vi "Image with metadata to Tiff file string.vi"(4 "error in":errorcluster, 5 "Compression Type (None)":i32(ring) items=["None", "JPEG", "Run Length Encoded", "Zip"], 6 "ImageDescription string\n(must be at least 5 char long)":string=" Four score and seven years ago our fathers brought forth on this continent, a new nation, conceived in Liberty, and dedicated to the proposition that all men are created equal.\n\nNow we are engaged in a great civil war, testing whether that nation, or any nation so conceived and so dedicated, can long endure. We are met on a great battle-field of that war. We have come to dedicate a portion of that field, as a final resting place for those who here gave their lives that that nation might live. It is altogether fitting and proper that we should do this.\n\nBut, in a larger sense, we can not dedicate -- we can not consecrate -- we can not hallow -- this ground. The brave men, living and dead, who struggled here, have consecrated it, far above our poor power to add or detract. The world will little note, nor long remember what we say here, but it can never forget what they did here. It is for us the living, rather, to be dedicated here to the unfinished work which they who fought here have thus far so nobly advanced. It is rather for us to be here dedicated to the great task remaining before us -- that from these honored dead we take increased devotion to that cause for which they gave the last full measure of devotion -- that we here highly resolve that these dead shall not have died in vain -- that this nation, under God, shall have a new birth of freedom -- and that government of the people, by the people, for the people, shall not perish from the earth. ", 7 "img":T1) -> (0 "error out":errorcluster, 1 "Time elapsed (ms)":u32, 2 "Tiff file out (unsigned byte array)":u8[](array[numeric]), 3 "Image Out (duplicate)":T1)   [LabVIEW 2013, in "Tiff reader.lvlib"]
doc: "This .vi converts an image to a tiff file string with the \"Custom Data\" strings attached to the images to the Tiff file metadata."
uses:
  Tiff reader.lvlib
  <vilib>/vision/Image Controls.llb/IMAQ Image.ctl
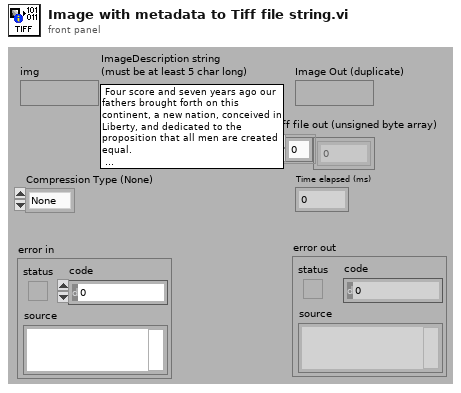
[diagram p1: front panel]
types:
  T1 = typedef "IMAQ Image.ctl" = refnum<image>
  T2 = cluster{"Rows Per Strip":i32, "Photometric":i32, "Compression Type":i32}
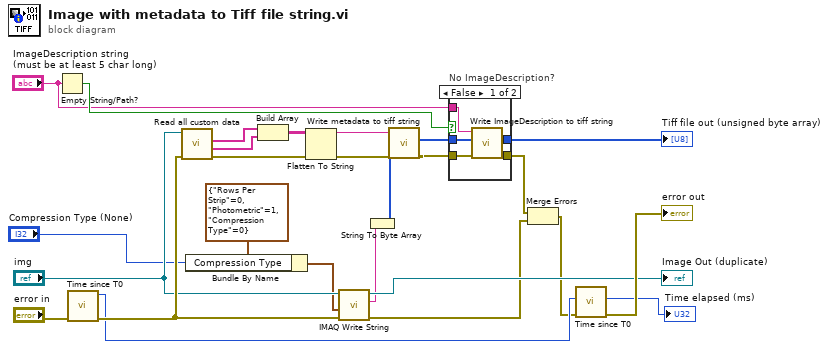
[diagram p0: block diagram]
diagram:
  n1 = Empty String/Path?(string/path="ImageDescription string\n(must be at least 5 char long)") -> (empty?=w4:bool)
  n2 = call "Time since T0.vi"("error in (no error)"="error in") -> ("error out"=w26:errorcluster, "current ms"=w14:u32)  [unwired: 2 in, 3 out]
  n3 = call "Read all custom data.vi"("error in (no error)"=w26, "img"="img") -> ("error out"=w16:errorcluster, "Custom Data"=w18:string[], "Keys"=w19:string[])  [unwired: 7 out]
  n4 = Bundle By Name(cluster=T2 {"Rows Per Strip"=0, "Photometric"=1, "Compression Type"=0} ("TIFF Options"), "Compression Type"="Compression Type (None)") -> (w9:T2)
  n5 = Build Array(w19, w18) -> (w17:string[][])
  n6 = Flatten To String(anything=w17, error in (no error)=w16) -> (data string=w20:string, error out=w24:errorcluster)  [unwired: 3 out]
  n7 = call-poly "IMAQ Write String"("error in (no error)"=w26, "TIFF Options"=w9, "Image"="img") -> ("error out"=w12:errorcluster, "FileString"=w21:string, "Image Out (duplicate)"=→"Image Out (duplicate)":T1)  [unwired: 2 in, 4 out]
  n8 = String To Byte Array(string=w21) -> (unsigned byte array=w1:u8[])
  n9 = call "Write metadata to tiff string.vi"("error in"=w24, "Tiff image (unsigned byte array)"=w1, "Metadata string\n(must be at least 5 char long)"=w20) -> ("error out"=w6:errorcluster, "Tiff file out (unsigned byte array)"=w5:u8[])  [unwired: 2 in, 5 out]
  n10 = case "No ImageDescription?" shown="False" w4 {
    tunnel: [w31 w33] -> w7
    tunnel: w6 -> [w30 w33]
    tunnel: w5 -> [w29 w32]
    tunnel: "ImageDescription string\n(must be at least 5 char long)" -> [w28 _]
    tunnel: [w27 w32] -> w2
    frame False {
      n11 = call "Write ImageDescription to tiff string.vi"("error in"=w30, "Tiff image (unsigned byte array)"=w29, "ImageDescription string\n(must be at least 5 char long)"=w28) -> ("error out"=w31:errorcluster, "Tiff file out (unsigned byte array)"=w27:u8[])  [unwired: 7 in]
    }
    frame True {
    }
  }
  "Tiff file out (unsigned byte array)" <- w2
  n12 = Merge Errors(w7, w12) -> (w11:errorcluster)
  n13 = call "Time since T0.vi"("error in (no error)"=w11, "T0 millisecond timer value"=w14) -> ("error out"=→"error out":errorcluster, "Time elapsed (ms)"=→"Time elapsed (ms)":u32)  [unwired: 1 in, 3 out]
